vi "Lockin_autoscale.vi"(3 "error in (no error)":errorcluster, 4 "Integration time (ms)":u32, 6 "VISA resource name":refnum<visa-resource-name>="GPIB0::7::INSTR") -> (0 "error out":errorcluster, 1 "String":string, 2 "VISA resource name out":refnum<visa-resource-name>="GPIB0::7::INSTR")   [LabVIEW 2023]
uses:
  Stanford Research 830/Public/Data/Read (1 Parameter).vi
  Stanford Research 830/Stanford Research 830.lvlib
panel:
  out "Times":i32
  # "How many times to check whether the setted sensitivity is appropriate before send it out."
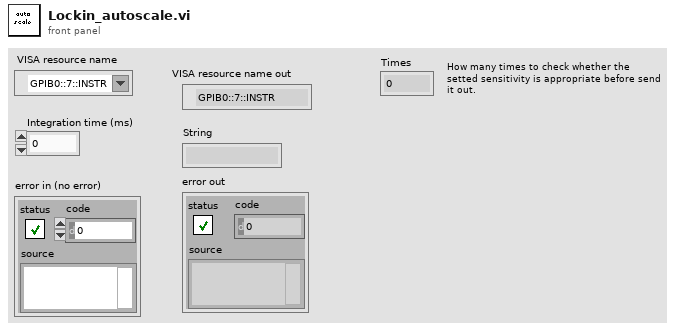
[diagram p1: front panel]
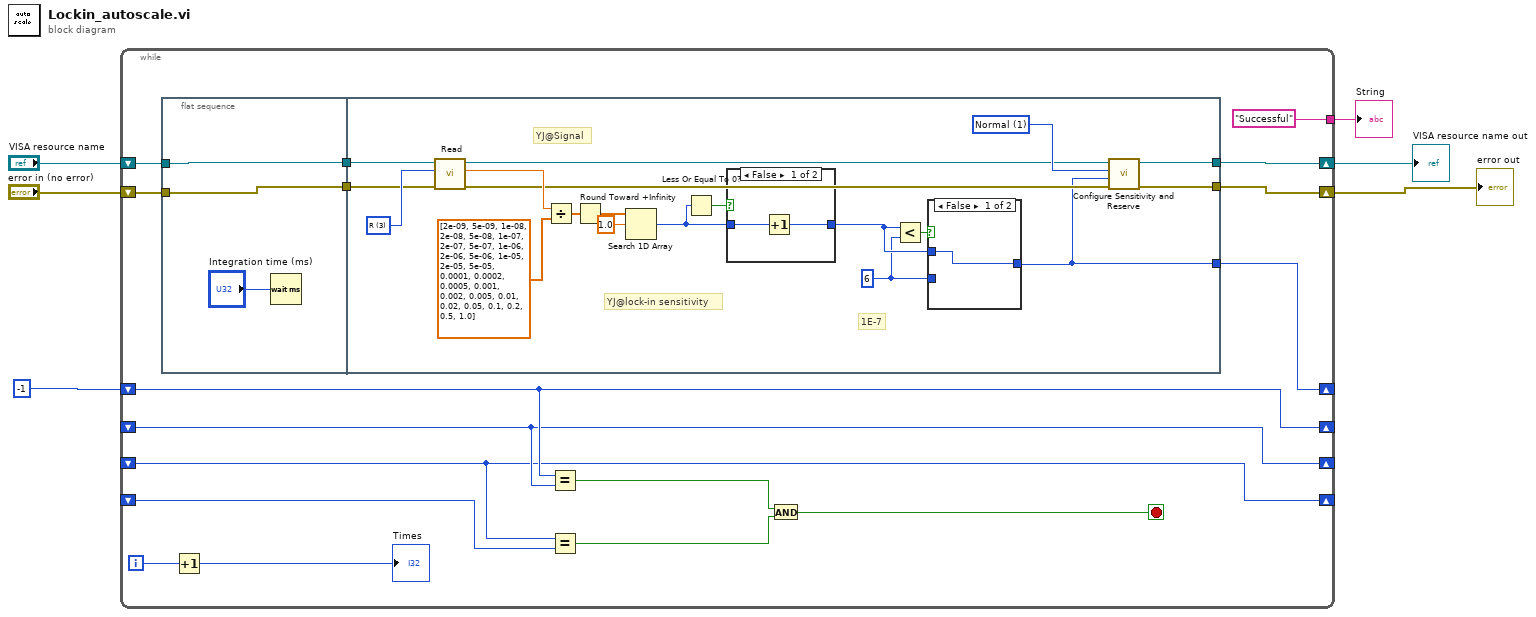
[diagram p0: block diagram]
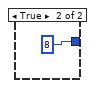
[diagram p3: hidden frame]
diagram:
  n1 = while {
    shift-right: [w19] -> w4
    shift-left: "VISA resource name" -> [w22]
    shift-right: [w18] -> w2
    shift-left: "error in (no error)" -> [w23]
    shift-right: [w17] -> _
    shift-left: -1 -> [w16]
    shift-right: [w16] -> _
    shift-left: _ -> [w15]
    shift-right: [w15] -> _
    shift-left: _ -> [w14]
    shift-right: [w14] -> _
    shift-left: _ -> [w13]
    tunnel: ["Successful" ("String")] -> w1
    i -> [w8]
    stop <- w10 stop-if-true
    n2 = flat-sequence {
      tunnel: [w26] -> w21
      tunnel: [w25] -> w20
      tunnel: w22 -> [w26]
      tunnel: w23 -> [w25]
      tunnel: w21 -> [w37]
      tunnel: w20 -> [w36]
      tunnel: [w32] -> w19
      tunnel: [w31] -> w18
      tunnel: [w29] -> w17
      frame #0 {
        n3 = Wait (ms)(milliseconds to wait="Integration time (ms)") -> ()  [unwired: 1 out]
      }
      frame #1 {
        w27 = 6 ("y")
        w38 = i16 1 items=["Auto Reserve"=-1, "High Reserve"=0, "Normal"=1, "Low Noise"=2] ("Dynamic Reserve (-1: Auto Reserve)")
        w45 = u16 3 items=["X"=1, "Y"=2, "R"=3, "Theta"=4, "Channel 1"=5, "Channel 2"=6, "Aux In 1"=7, "Aux In 2"=8, "Aux In 3"=9, "Aux In 4"=10] ("Parameter (1: X)")
        # "1E-7"
        # "YJ@Signal"
        # "YJ@lock-in sensitivity"
        n4 = call-poly "Read.vi"("error in (no error)"=w36, "Parameter (1: X)"=w45, "VISA resource name"=w37) -> ("error out"=w33:errorcluster, "Measurement"=w35:dbl, "VISA resource name out"=w34:refnum<visa-resource-name>)  [unwired: 6 in]
        n5 = Divide(x=w35, y=dbl[] [2e-09, 5e-09, 1e-08, 2e-08, 5e-08, 1e-07, 2e-07, 5e-07, 1e-06, 2e-06, 5e-06, 1e-05, 2e-05, 5e-05, 0.0001, 0.0002, 0.0005, 0.001, 0.002, 0.005, 0.01, 0.02, 0.05, 0.1, 0.2, 0.5, 1.0]) -> (x/y=w39:dbl[])
        n6 = Round Toward +Infinity(x=w39) -> (ceil(x): smallest int >= x=w40:dbl[])
        n7 = Search 1D Array(1D array=w40, element=1.0) -> (index of element=w43:i32)  [unwired: 1 in]
        n8 = Less Or Equal To 0?(x=w43) -> (x <= 0?=w42:bool)
        n9 = case shown="False" w42 {
          tunnel: [w48 8] -> w28
          tunnel: w43 -> [w49 _]
          frame False {
            n10 = Increment(x=w49) -> (x+1=w48:i32)
          }
          frame True {
          }
        }
        n11 = Less?(x=w28, y=w27) -> (x < y?=w30:bool)
        n12 = case shown="False" w30 {
          tunnel: [w46 w47] -> w29
          tunnel: w27 -> [_ w47]
          tunnel: w28 -> [w46 _]
          frame False {
          }
          frame True {
          }
        }
        n13 = call "Configure Sensitivity and Reserve.vi"("error in (no error)"=w33, "Sensitivity (-1: Auto gain)"=w29, "Dynamic Reserve (-1: Auto Reserve)"=w38, "VISA resource name"=w34) -> ("error out"=w31:errorcluster, "VISA resource name out"=w32:refnum<visa-resource-name>)  [unwired: 6 in]
      }
    }
    n14 = Increment(x=w8) -> (x+1=→"Times":i32)
    n15 = Equal?(x=w16, y=w15) -> (x = y?=w12:bool)
    n16 = Equal?(x=w14, y=w13) -> (x = y?=w11:bool)
    n17 = And(x=w12, y=w11) -> (x .and. y?=w10:bool)
  }
  "error out" <- w2
  "VISA resource name out" <- w4
  "String" <- w1
